vi "Init stream.vi"(8 "min sample rate":dbl=97000000.0 format="%.2p", 9 "channel name":string="0,2", 10 "SCOPE Resource":refnum<k15>="Dev1" caption="NI-Scope Resource", 11 "FPGA VI Reference":T1) -> (0 "error out":errorcluster, 1 "stream session":refnum<k20>, 2 "instrument handle out":refnum<k15>, 3 "FPGA VI Reference out":T1, 5 "Actual Sample Rate":dbl)   [LabVIEW 2013]
uses:
  fpga_ref_minimal.ctl
  <instrlib>/niScope/Controls/niScope vertical coupling.ctl
  <instrlib>/niScope/Controls/niScope trigger slope.ctl
  <instrlib>/niScope/Controls/niScope trigger source digital.ctl
  <instrlib>/niScope/Configure/Trigger/niScope Configure Trigger Digital.vi
  <vilib>/FPGAPlugInAG/Dynamic/niLvFpga_P2PGetEndpoint_Dynamic.vi
  <vilib>/rvi/interface/nirviMethod/nirviMethod.xnode
  <vilib>/rvi/errors/niLvFpgaMergeErrorWithErrorCode.vi
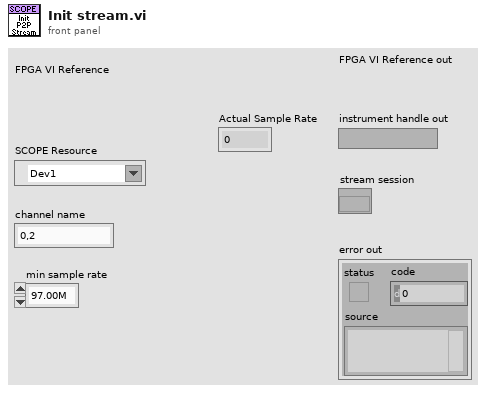
[diagram p1: front panel]
types:
  T1 = typedef "fpga_ref_minimal.ctl" = refnum<k20>
  T2 = typedef "niScope trigger source digital.ctl" = string
  T3 = typedef "niScope trigger slope.ctl" = i32
  T4 = typedef "niScope vertical coupling.ctl" = i32
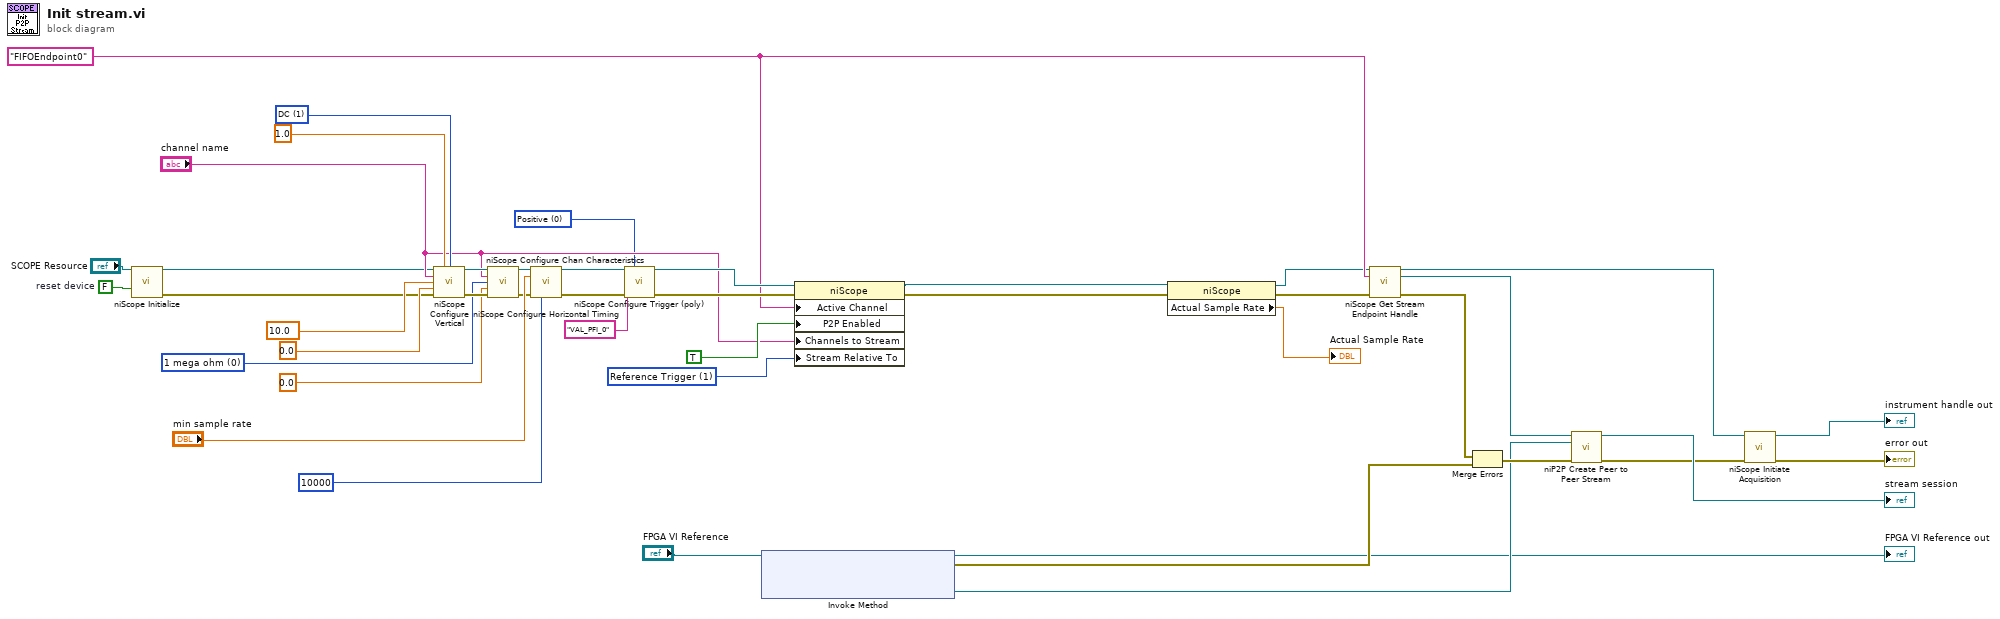
[diagram p0: block diagram]
diagram:
  w2 = T3 0 items=["Positive", "Negative"] ("trigger slope")
  w3 = 1 items=["Start Trigger", "Reference Trigger", "Sync Trigger"] ("Peer-to-Peer:Stream Relative To")
  w33 = u32 0 items=["1 mega ohm"=0, "50 ohms"=2] ("input impedance")
  w31 = T4 1 items=["AC", "DC", "Ground"] ("vertical coupling")
  w16 = "FIFOEndpoint0" ("Active Channel")
  w43 = FALSE  # reset device
  n1 = call <instrlib>:"niScope Initialize.vi"("resource name"="SCOPE Resource", "reset device"=w43) -> ("instrument handle"=w14:refnum<k15>, "error out"=w13:errorcluster)  [unwired: 12 in]
  n2 = call <instrlib>:"niScope Configure Vertical.vi"("instrument handle"=w14, "probe attenuation"=1.0, "vertical coupling"=w31, "channels"="channel name", "vertical range"=10.0, "vertical offset"=0.0, "error in"=w13) -> ("instrument handle out"=w39:refnum<k15>, "error out"=w38:errorcluster)  [unwired: 7 in]
  n3 = call <instrlib>:"niScope Configure Chan Characteristics.vi"("instrument handle"=w39, "channels"="channel name", "input impedance"=w33, "maximum input frequency"=0.0, "error in"=w38) -> ("instrument handle out"=w36:refnum<k15>, "error out"=w37:errorcluster)  [unwired: 9 in]
  n4 = call <instrlib>:"niScope Configure Horizontal Timing.vi"("instrument handle"=w36, "min sample rate"="min sample rate", "error in"=w37, "min record length"=10000) -> ("instrument handle out"=w19:refnum<k15>, "error out"=w18:errorcluster)  [unwired: 10 in]
  n5 = call-poly <instrlib>:"niScope Configure Trigger (poly).vi"("instrument handle"=w19, "trigger slope"=w2, "trigger source"=T2 "VAL_PFI_0", "error in"=w18) -> ("instrument handle out"=w30:refnum<k15>, "error out"=w29:errorcluster)  [unwired: 10 in]
  n6 = xnode "Invoke Method"("FPGA VI Reference In"="FPGA VI Reference") -> ("FPGA VI Reference Out"=→"FPGA VI Reference out":T1, "error out"=w24:errorcluster, "Reader"=w25:refnum<k20>)  [unwired: 1 in]
  n7 = property class="niScope"(reference=w30, error in=w29, "Active Channel"=w16, "P2P Enabled"=TRUE ("Peer-to-Peer:P2P Enabled"), "Channels to Stream"="channel name", "Stream Relative To"=w3) -> (reference out=w5:refnum<k15>, error out=w9:errorcluster)
  n8 = property class="niScope"(reference=w5, error in=w9) -> (reference out=w7:refnum<k15>, error out=w8:errorcluster, "Actual Sample Rate"=→"Actual Sample Rate":dbl)
  n9 = call <instrlib>:"niScope Get Stream Endpoint Handle.vi"("instrument handle"=w7, "stream endpoint"=w16, "error in"=w8) -> ("instrument handle out"=w21:refnum<k15>, "writer handle"=w12:refnum<k20>, "error out"=w27:errorcluster)  [unwired: 10 in]
  n10 = Merge Errors(w27, w24) -> (w28:errorcluster)
  n11 = call <vilib>:"niP2P Create Peer to Peer Stream.vi"("writer"=w12, "reader"=w25, "error in (no error)"=w28) -> ("stream session"=→"stream session":refnum<k20>, "error out"=w10:errorcluster)  [unwired: 11 in]
  n12 = call <instrlib>:"niScope Initiate Acquisition.vi"("instrument handle"=w21, "error in"=w10) -> ("instrument handle out"=→"instrument handle out":refnum<k15>, "error out"=→"error out":errorcluster)  [unwired: 12 in]
